vi "SimplePidController (SubVI).vi"(9 "Encoder Count Difference":i32, 10 "Period of Timed Loop":dbl, 11 "Speed Setpoint":dbl(slide) scale=-1.6..1.6) -> (1 "Output to Duty Cycle":dbl, 2 "Output to PWM":dbl format="%.2f", 3 "Speed of Motor":dbl, 4 "Boolean Output for Motor Driver":bool)   [LabVIEW 2017]
uses:
  <vilib>/addons/control/pid/pid.llb/PID (DBL).vi
  <vilib>/addons/control/pid/NI_PID_pid.lvlib
panel:
  # "VI Name: SimplePidController (SubVI).vi\nAuthor: Steven Lee\n\nThis SubVI takes in the Encoder Count Difference and provides PID control for the robot.\nPlease see the block diagram for more details."
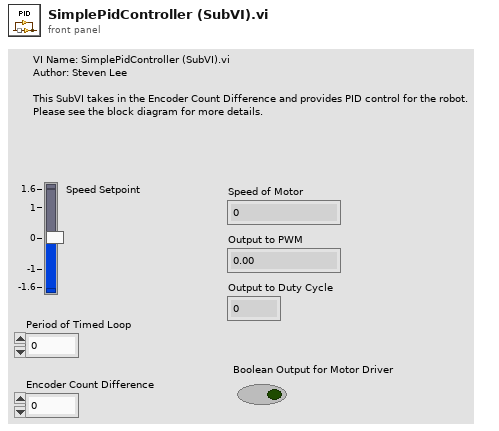
[diagram p1: front panel]
types:
  T1 = cluster{"proportional gain (Kc)":dbl, "integral time (Ti, min)":dbl, "derivative time (Td, min)":dbl}
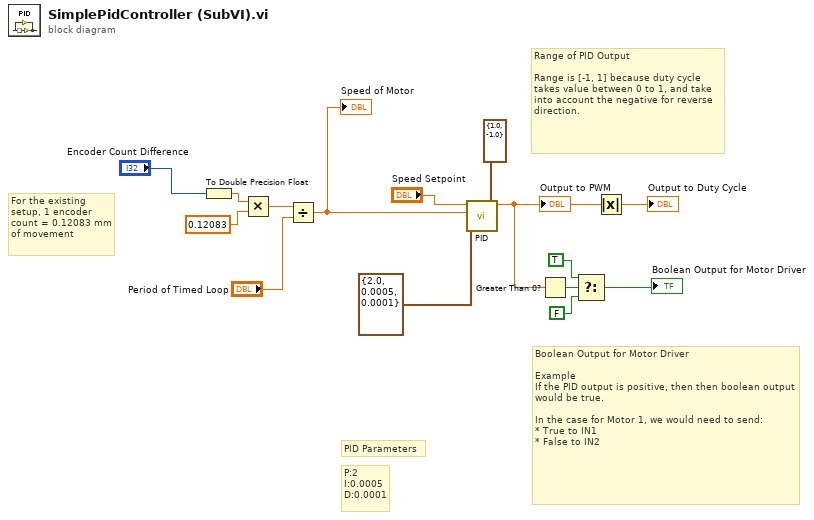
[diagram p0: block diagram]
diagram:
  # "P:2\nI:0.0005\nD:0.0001"
  # "Boolean Output for Motor Driver\n\nExample\nIf the PID output is positive, then then boolean output would be true.\n\nIn the case for Motor 1, we would need to send:\n* True to IN1\n* False to IN2"
  # "Range of PID Output\n\nRange is [-1, 1] because duty cycle takes value between 0 to 1, and take into account the negative for reverse direction."
  # "PID Parameters"
  # "For the existing setup, 1 encoder count = 0.12083 mm of movement"
  n1 = To Double Precision Float(number="Encoder Count Difference") -> (double precision float=w1:dbl)
  n2 = Multiply(x=w1, y=0.12083) -> (x*y=w3:dbl)
  n3 = Divide(x=w3, y="Period of Timed Loop") -> (x/y=w6:dbl)
  "Speed of Motor" <- w6
  n4 = call-poly <vilib>:"PID.vi"("output range"=cluster{"output high":dbl, "output low":dbl} {"output high"=1.0, "output low"=-1.0}, "PID gains"=T1 {"proportional gain (Kc)"=2.0, "integral time (Ti, min)"=0.0005, "derivative time (Td, min)"=0.0001}, "process variable"=w6, "setpoint"="Speed Setpoint") -> ("output"=w8:dbl)  [unwired: 6 in, 1 out]
  "Output to PWM" <- w8
  n5 = Greater Than 0?(x=w8) -> (x > 0?=w9:bool)
  n6 = Select(t=TRUE, s=w9, f=FALSE) -> (s? t:f=→"Boolean Output for Motor Driver":bool)
  n7 = Absolute Value(x=w8) -> (abs(x)=→"Output to Duty Cycle":dbl)
